vi "FTW-CodeGen-FindTerm-Variant.vi"(5 "Terminals":cluster{"Type":variant, "ID":string}[](array[cluster]), 7 "Terminal ID":string) -> (6 "Terminal Type":variant, 8 "Found?":bool)   [LabVIEW 2015]
panel:
  # "Inputs"
  # "Outputs"
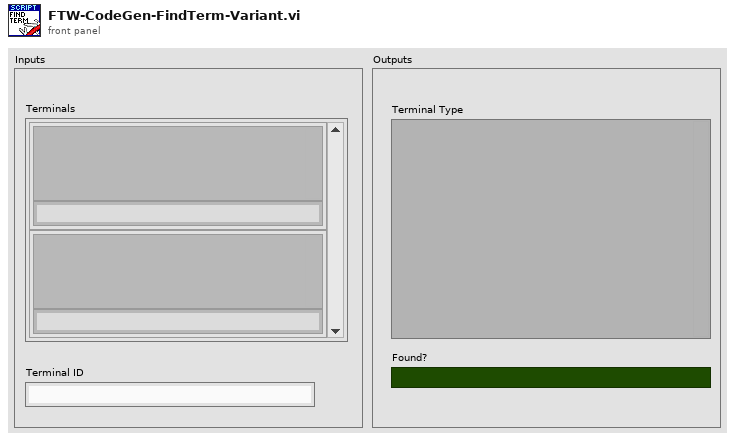
[diagram p1: front panel]
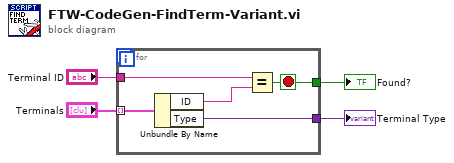
[diagram p0: block diagram]
diagram:
  n1 = for {
    tunnel: [w9] -> w1
    tunnel: [w8] -> w4
    tunnel: "Terminals" -> [w7] mode=indexing
    tunnel: "Terminal ID" -> [w5]
    stop <- w8 stop-if-true
    n2 = Unbundle By Name(w7) -> ("ID"=w6:string, "Type"=w9:variant)
    n3 = Equal?(x=w5, y=w6) -> (x = y?=w8:bool)
  }
  "Terminal Type" <- w1
  "Found?" <- w4
